vi "Data Plotter.vi"() -> ()   [LabVIEW 2016]
uses:
  Type Defs/Boxcar.ctl
  Type Defs/Sensor Data.ctl
panel:
  out "TC Array":dbl[](array[numeric])=[22.795104477500004, 29.692077105500005, 29.791259233999995, 29.692077105500005, 29.890441362500013, 29.791259233999995, 29.791259233999995, 22.383899999999997, 1369.6815, 1369.6815, 1369.6815, 1369.6815, 1369.6815, 1369.6815]
  out "?":T1(graph)={"TC Array[0]"=22.795104477500004, "TC Array[1]"=29.692077105500005, "TC Array[2]"=29.791259233999995, "TC Array[3]"=29.692077105500005, "TC Array[4]"=29.890441362500013, "TC Array[5]"=29.791259233999995, "TC Array[6]"=29.791259233999995, "TC Array[7]"=22.383899999999997, "TC Array[8]"=1369.6815, "TC Array[9]"=1369.6815, "TC Array[10]"=1369.6815, "TC Array[11]"=1369.6815, "TC Array[12]"=1369.6815, "TC Array[13]"=1369.6815}
  out "Array":string[](array[string])=["-1.63", "-1.92", "-1.17", "-3.66", "-7.67", "-1.53", "-1.53", "-6.64", "-1.03", "-1.67", "0.00", "0.00", "0.00", "0.00", "0.00", "0.00", "-10.00", "-10.00", "-10.00", "-10.00", "-83333.00", "-83333.30", "0.00", "0.00", "0.00", "0.00", "0.00", "0.00", "0.00", "0.00", "0.00", "0.00"]
  out "?":T2(graph)={"[0]"=-1.63, "[1]"=-1.92, "[2]"=-1.17, "[3]"=-3.66, "[4]"=-7.67, "[5]"=-1.53, "[6]"=-1.53, "[7]"=-6.64, "[8]"=-1.03, "[9]"=-1.67, "[10]"=0.0, "[11]"=0.0, "[12]"=0.0, "[13]"=0.0, "[14]"=0.0, "[15]"=0.0, "[16]"=-10.0, "[17]"=-10.0, "[18]"=-10.0, "[19]"=-10.0, "[20]"=-83333.0, "[21]"=-83333.3, "[22]"=0.0, "[23]"=0.0}
  in  "stop":bool
  # "CSULB Launch Team Control System"
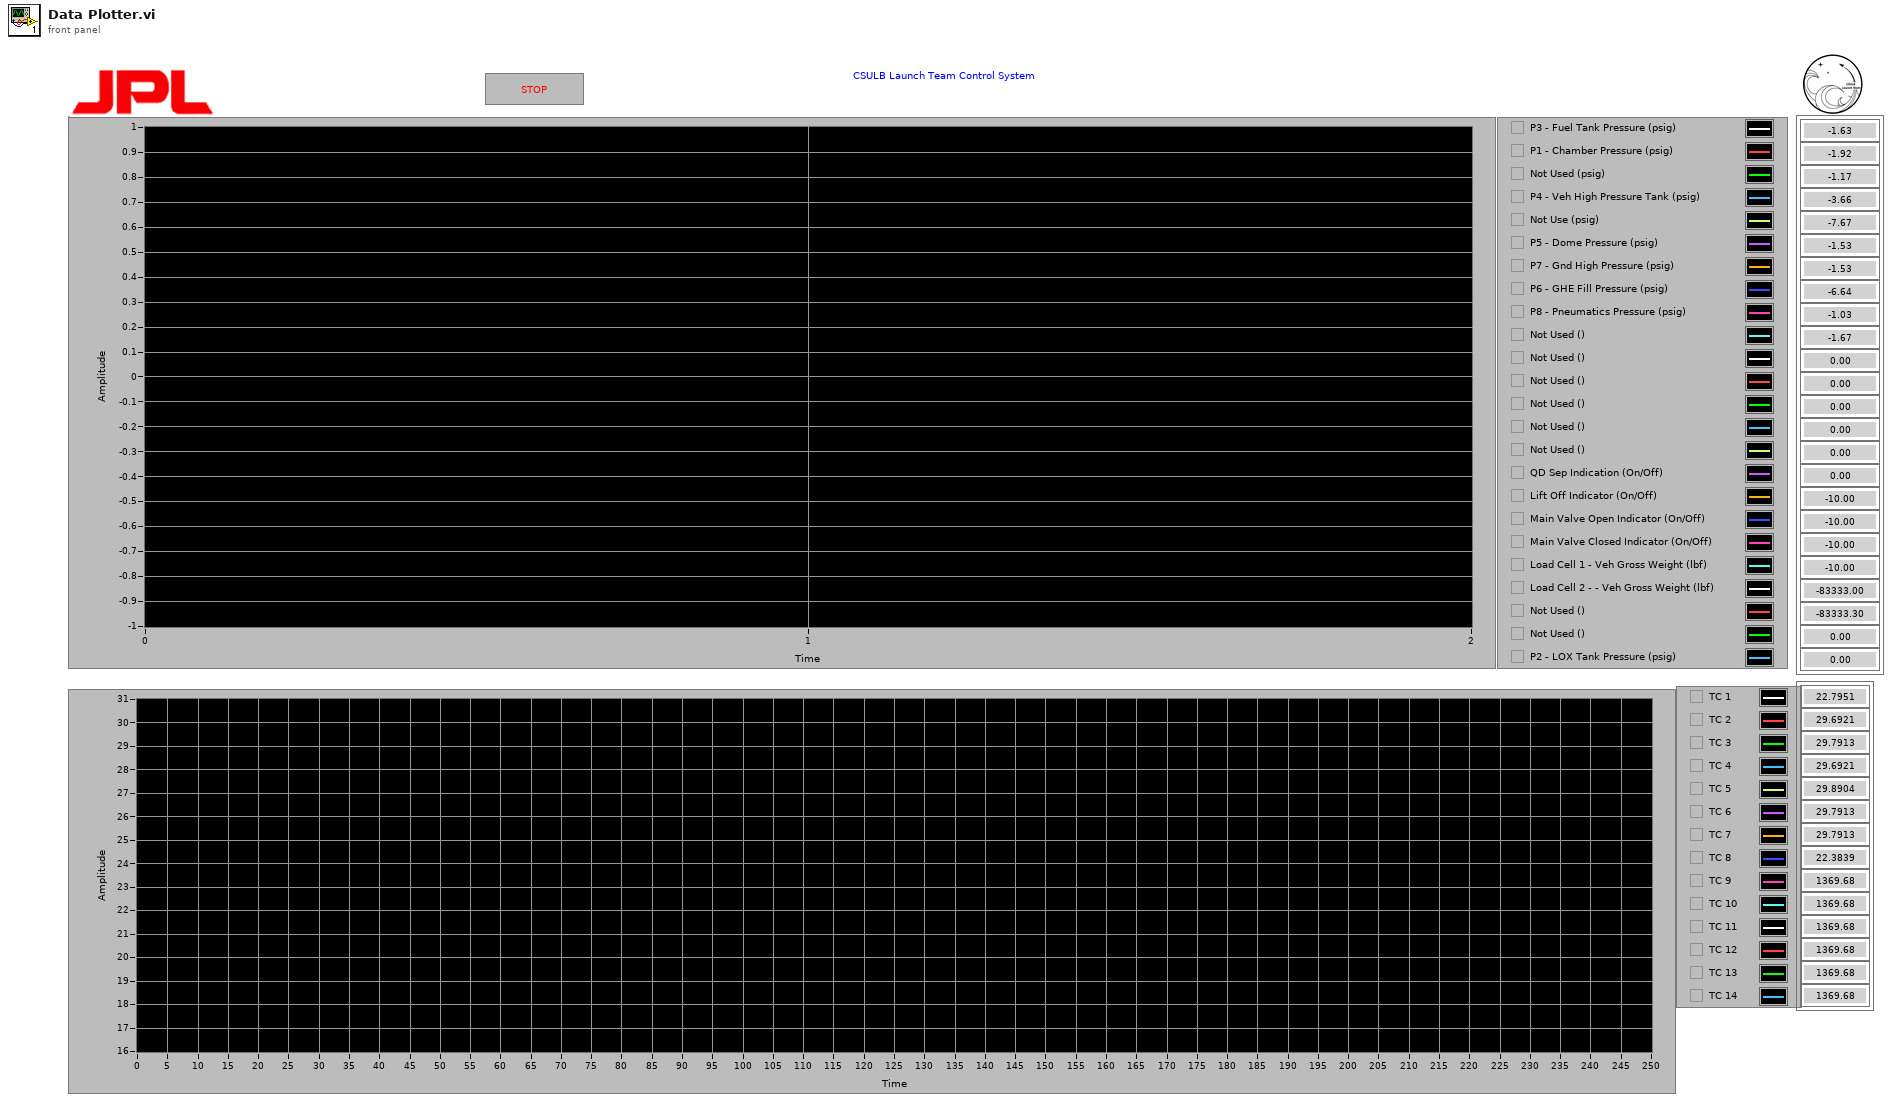
[diagram p1: front panel]
types:
  T1 = cluster{"TC Array[0]":dbl, "TC Array[1]":dbl, "TC Array[2]":dbl, "TC Array[3]":dbl, "TC Array[4]":dbl, "TC Array[5]":dbl, "TC Array[6]":dbl, "TC Array[7]":dbl, "TC Array[8]":dbl, "TC Array[9]":dbl, "TC Array[10]":dbl, "TC Array[11]":dbl, "TC Array[12]":dbl, "TC Array[13]":dbl}
  T2 = cluster{"[0]":dbl, "[1]":dbl, "[2]":dbl, "[3]":dbl, "[4]":dbl, "[5]":dbl, "[6]":dbl, "[7]":dbl, "[8]":dbl, "[9]":dbl, "[10]":dbl, "[11]":dbl, "[12]":dbl, "[13]":dbl, "[14]":dbl, "[15]":dbl, "[16]":dbl, "[17]":dbl, "[18]":dbl, "[19]":dbl, "[20]":dbl, "[21]":dbl, "[22]":dbl, "[23]":dbl}
  T3 = typedef "Boxcar.ctl" = cluster{"AI Sensor Data":T4, "TC Array":dbl[]}
  T4 = typedef "Sensor Data.ctl" = cluster{"Sensor Array":cluster{"Description":string, "Last Reading":string, "Coefs":dbl[], "Eng Units":string}[]}
  T5 = cluster{"Description":string, "Last Reading":string, "Coefs":dbl[], "Eng Units":string}[]
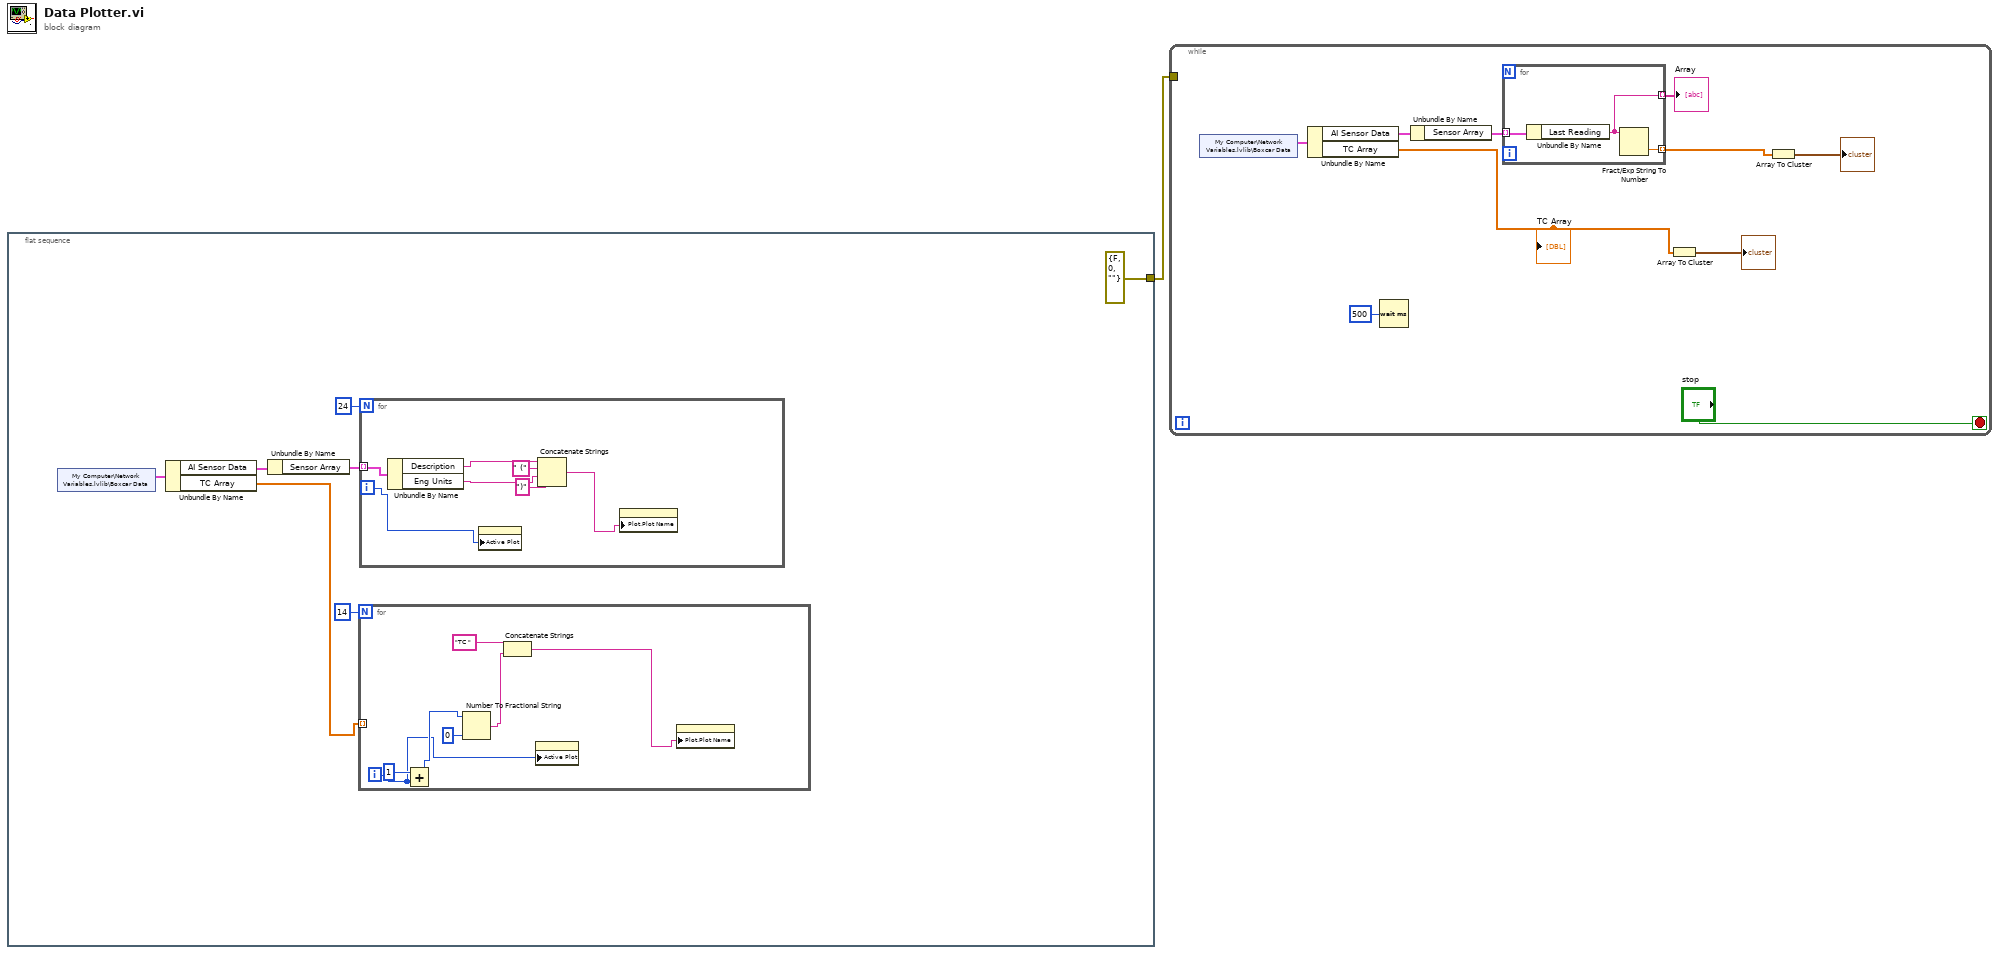
[diagram p0: block diagram]
diagram:
  n1 = flat-sequence {
    tunnel: [errorcluster {"status"=FALSE, "code"=0, "source"=""} ("error constant")] -> w1
    frame #0 {
      n2 = shared-variable "My Computer\\Network Variables.lvlib\\Boxcar Data"() -> (w5:T3)  [unwired: 1 in, 1 out]
      n3 = Unbundle By Name(w5) -> ("AI Sensor Data"=w6:T4, "TC Array"=w4:dbl[])
      n4 = Unbundle By Name(w6) -> ("Sensor Array"=w7:T5)
      n5 = for {
        N: 14 -> [_]
        tunnel: w4 -> [_] mode=indexing
        i -> [w9]
        n6 = Add(x=1, y=w9) -> (x+y=w14:i32)
        n7 = Number To Fractional String(number=w14, precision (6)=i16 0) -> (F-format string=w11:string)  [unwired: 2 in]
        n8 = Concatenate Strings("TC ", w11) -> (w10:string)
        n9 = property class="WFChart (strict)"("Active Plot"=w9) -> ()  [unwired: 2 in, 2 out]
        n10 = property class="WFChart (strict)"("Plot.Plot Name"=w10) -> ()  [unwired: 2 in, 2 out]
      }
      n11 = for {
        N: 24 -> [_]
        tunnel: w7 -> [w22] mode=indexing
        i -> [w17]
        n12 = Unbundle By Name(w22) -> ("Description"=w21:string, "Eng Units"=w19:string)
        n13 = property class="WFChart (strict)"("Active Plot"=w17) -> ()  [unwired: 2 in, 2 out]
        n14 = Concatenate Strings(w21, " (" ("string"), w19, ")" ("string")) -> (w16:string)
        n15 = property class="WFChart (strict)"("Plot.Plot Name"=w16) -> ()  [unwired: 2 in, 2 out]
      }
    }
  }
  n16 = while {
    tunnel: w1 -> [_]
    stop <- "stop" stop-if-true
    n17 = shared-variable "My Computer\\Network Variables.lvlib\\Boxcar Data"() -> (w31:T3)  [unwired: 1 in, 1 out]
    n18 = Unbundle By Name(w31) -> ("AI Sensor Data"=w30:T4, "TC Array"=w24:dbl[])
    "TC Array" <- w24
    n19 = Wait (ms)(milliseconds to wait=u32 500) -> ()  [unwired: 1 out]
    n20 = Unbundle By Name(w30) -> ("Sensor Array"=w29:T5)
    n21 = for {
      tunnel: w29 -> [w35] mode=indexing
      tunnel: [w34] -> w28 mode=indexing
      tunnel: [w33] -> w26 mode=indexing
      n22 = Unbundle By Name(w35) -> ("Last Reading"=w33:string)
      n23 = Fract/Exp String To Number(string=w33) -> (number=w34:dbl)  [unwired: 3 in, 1 out]
    }
    "Array" <- w26
    n24 = Array To Cluster(array=w24) -> (cluster=→"?":T1)
    n25 = Array To Cluster(array=w28) -> (cluster=→"?":T2)
  }
